vi "front.vi"(7 "Parâmetros Ini 2":T2={"Gyro Port"=0, "Sensor - Left"=3, "Sensor - Right"=2, "     Color \nSensor Port"=1, "Kp Front"=0.5, "Motor speed"=-15, "Distance to street"=0.0, "Motor speed turns"=16, "Kp Curvas"=0.0} {"Kp Front" format="%.3f"; "Color \nSensor Port" items=["Port 1", "Port 2", "Port 3", "Port 4"]; "Sensor - Right" items=["Port 1", "Port 2", "Port 3", "Port 4"]; "Sensor - Left" items=["Port 1", "Port 2", "Port 3", "Port 4"]; "Gyro Port" items=["Port 1", "Port 2", "Port 3", "Port 4"]}, 8 "NXT/EV3":T1, 9 "Integral IN":dbl, 11 "First Angle":sgl) -> (0 "Integral OUT":dbl, 1 "NXT/EV3 2":T1)   [LabVIEW 2016]
uses:
  <vilib>/NXT/Subs/LVHSConnector.ctl
  <vilib>/NXT/LegoClasses/BrickReference/BrickReference.lvclass
  parametros.ctl
  <vilib>/NXT/Block Support/NXT_InputPort.ctl
  <vilib>/NXT/Block Support/NXT_OutputPort.ctl
  <vilib>/NXT/Dual Mode Library/Sensors/EV3_Gyro_Angle.vi
  <vilib>/NXT/Dual Mode Library/Display/drawNumber_float.vi
  <vilib>/NXT/NXTIO Xnodes/NXTIONodeSubVIs/NXTMoveMotors.vi
  <vilib>/NXT/NXTIO Xnodes/AddressXNode/NXTIOAddress.xnode
  <vilib>/NXT/NXTIO Xnodes/NXTIOXNode/NXTIO.xnode
panel:
  out "Degrees 2":sgl
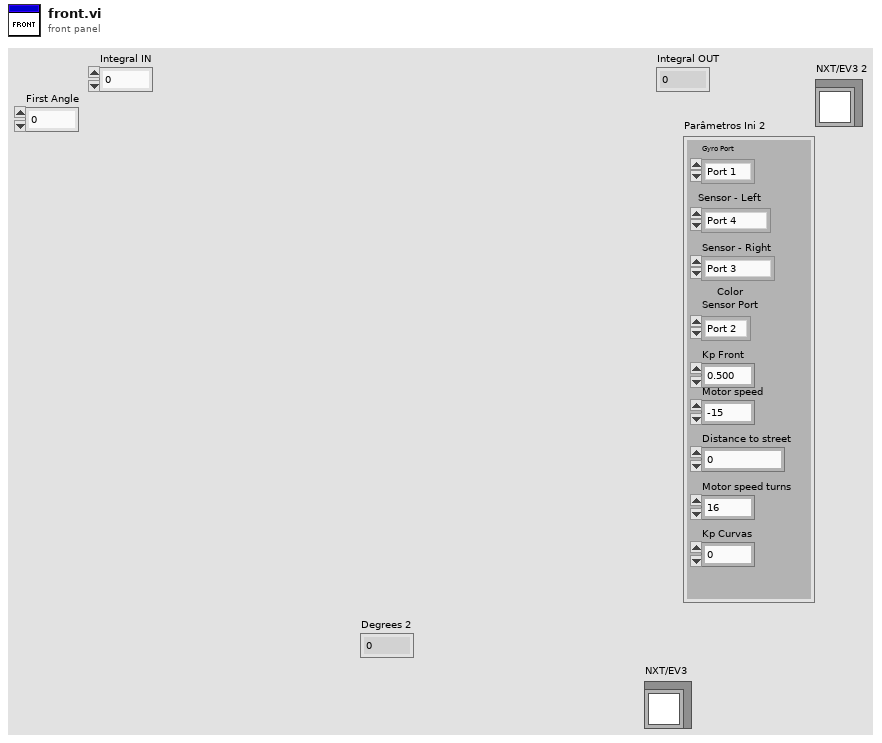
[diagram p1: front panel]
types:
  T1 = typedef "LVHSConnector.ctl" = refnum<class "BrickReference.lvclass">
  T2 = typedef "parametros.ctl" = cluster{"Gyro Port":T3, "Sensor - Left":T3, "Sensor - Right":T3, "     Color \nSensor Port":T3, "Kp Front":dbl, "Motor speed":i32, "Distance to street":dbl, "Motor speed turns":i32, "Kp Curvas":dbl}
  T3 = typedef "NXT_InputPort.ctl" = u32
  T4 = typedef "NXT_OutputPort.ctl" = u8
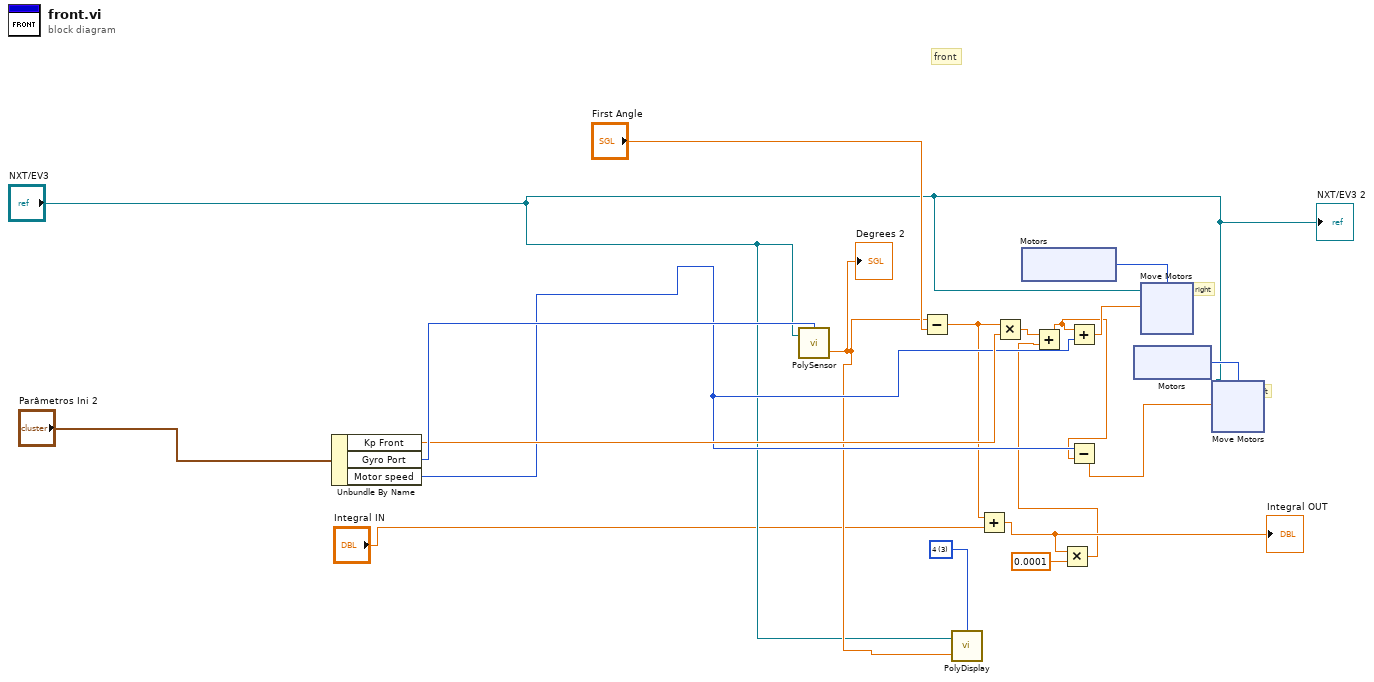
[diagram p0: block diagram]
diagram:
  w10 = i16 3 items=["1", "2", "3", "4", "5", "6", "7", "8", "9", "10", "11", "12"] ("Line")
  # "left"
  # "right"
  # "front"
  n1 = Unbundle By Name("Parâmetros Ini 2") -> ("Kp Front"=w13:dbl, "Gyro Port"=w19:T3, "Motor speed"=w11:i32)
  n2 = call-poly <vilib>:"PolySensor.vi"("NXT/EV3"="NXT/EV3", "Port (Port 1)"=w19) -> ("Degrees"=w9:sgl)  [unwired: 1 in, 1 out]
  "Degrees 2" <- w9
  n3 = Subtract(x=w9, y="First Angle") -> (x-y=w6:sgl)
  n4 = call-poly <vilib>:"PolyDisplay.vi"("number"=w9, "NXT/EV3"="NXT/EV3", "Line"=w10) -> ()  [unwired: 1 in, 1 out]
  n5 = Add(x=w6, y="Integral IN") -> (x+y=w4:dbl)
  "Integral OUT" <- w4
  n6 = Multiply(x=w6, y=w13) -> (x*y=w3:dbl)
  n7 = xnode "Motors"() -> ("Motor"=w16:T4)
  n8 = Multiply(x=w4, y=0.0001) -> (x*y=w2:dbl)
  n9 = Add(x=w3, y=w2) -> (x+y=w1:dbl)
  n10 = Add(x=w1, y=w11) -> (x+y=w18:dbl)
  n11 = Subtract(x=w11, y=w1) -> (x-y=w17:dbl)
  n12 = xnode "Motors"() -> ("Motor"=w15:T4)
  n13 = xnode "Move Motors"("Power/Speed 1"=w18, "Motors"=w16, "NXT/EV3"="NXT/EV3") -> ()  [unwired: 1 out]
  n14 = xnode "Move Motors"("Power/Speed 1"=w17, "Motors"=w15, "NXT/EV3"="NXT/EV3") -> ()  [unwired: 1 out]
  "NXT/EV3 2" <- "NXT/EV3"
